vi "From Datum Cluster.vi"(0 "Pair":T1) -> (2 "Map":refnum<class "Map.lvclass">)   [LabVIEW 2018, in "Toolkit.lvlib" / "Types.lvlib" / "Map.lvclass"]
uses:
  Map.lvclass
  Abstract/Abstract.lvclass
  Map.lvclass/Map.ctl
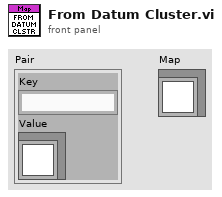
[diagram p1: front panel]
types:
  T1 = cluster{"Key":string, "Value":refnum<class "Abstract.lvclass">}
  T2 = cluster{"Key":string, "Value":refnum<class "Abstract.lvclass">}[]
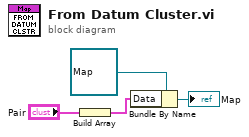
[diagram p0: block diagram]
diagram:
  n1 = Build Array("Pair") -> (w2:T2)
  n2 = Bundle By Name(cluster=refnum<class "Map.lvclass"> refnum ("Toolkit.lvlib:Data.lvlib:Map.lvclass"), "Data"=w2) -> (→"Map":refnum<class "Map.lvclass">)
